vi "Write Serial One by One With Echo.vi"(7 "String":string, 8 "Error In":errorcluster, 11 "VISA In":refnum<visa-resource-name>) -> (0 "Error Out":errorcluster, 3 "VISA Out":refnum<visa-resource-name>)   [LabVIEW 2017]
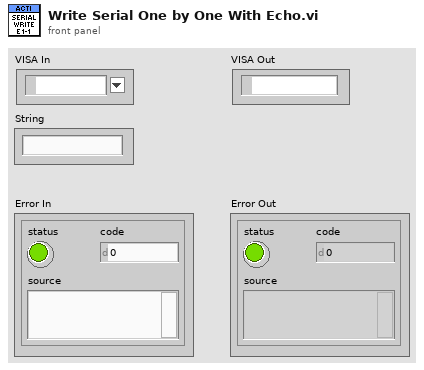
[diagram p1: front panel]
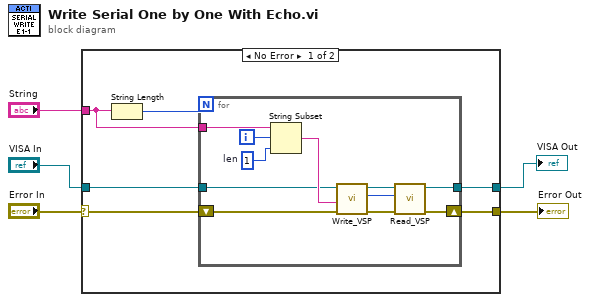
[diagram p0: block diagram]
diagram:
  n1 = case shown="No Error" "Error In" {
    selector: "Error In" -> [w11 w24]
    tunnel: [w10 w24] -> w4
    tunnel: "String" -> [w8 _]
    tunnel: "VISA In" -> [w7 w23]
    tunnel: [w6 w23] -> w1
    frame No Error {
      n2 = String Length(string=w8) -> (length=w9:i32)
      n3 = for {
        N: w9 -> [_]
        shift-right: [w17] -> w10
        shift-left: w11 -> [w19]
        tunnel: w8 -> [w20]
        tunnel: w7 -> [w15]
        tunnel: [w13] -> w6
        i -> [w22]
        w21 = 1  # len
        n4 = String Subset(string=w20, offset (0)=w22, length (rest)=w21) -> (substring=w16:string)
        n5 = call "Write_VSP.vi"("error in"=w19, "String"=w16, "VISA resource name"=w15) -> ("error out"=w18:errorcluster, "return count"=w12:u32, "duplicate VISA resource name"=w14:refnum<visa-resource-name>)  [unwired: 2 in]
        n6 = call "Read_VSP.vi"("error in"=w18, "Requested byte cout"=w12, "VISA resource name"=w14) -> ("error out"=w17:errorcluster, "duplicate VISA resource name"=w13:refnum<visa-resource-name>)  [unwired: 1 in, 2 out]
      }
    }
    frame Error {
    }
  }
  "Error Out" <- w4
  "VISA Out" <- w1
